vi "common_GUI_UpdateDeviceList.vi"(8 "error in (no error)":errorcluster, 9 "Controls[]":refnum<vi>[](array[refnum]), 10 "Arguments":string, 11 "SQL Server Info":T2) -> (0 "error out":errorcluster)   [LabVIEW 2013]
uses:
  Shared/MySQL/typedefs/mysql_authentication.ctl
panel:
  out "Array":string[](array[string])
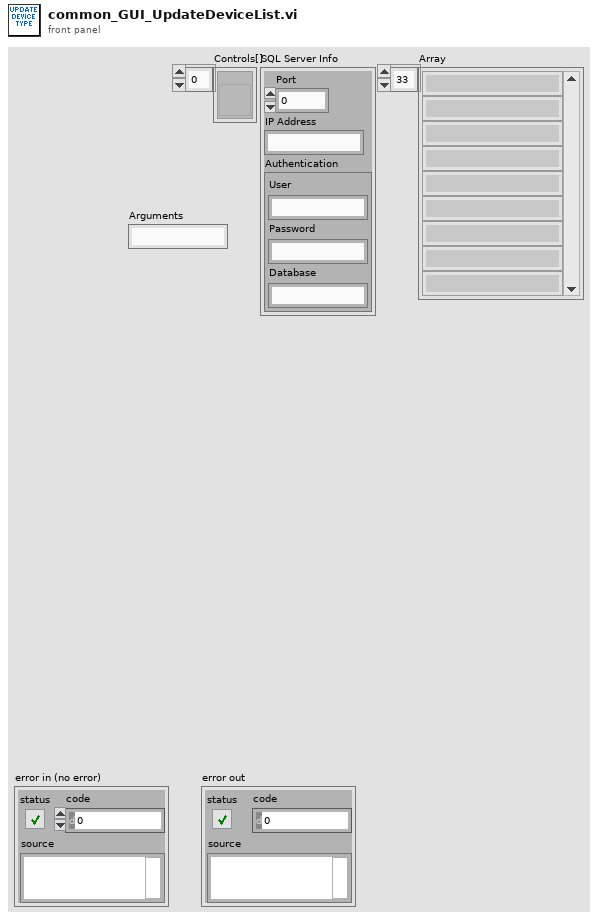
[diagram p1: front panel]
types:
  T1 = typedef "mysql_authentication.ctl" = cluster{"User":string, "Password":string, "Database":string}
  T2 = cluster{"Port":u16, "IP Address":string, "Authentication":T1}
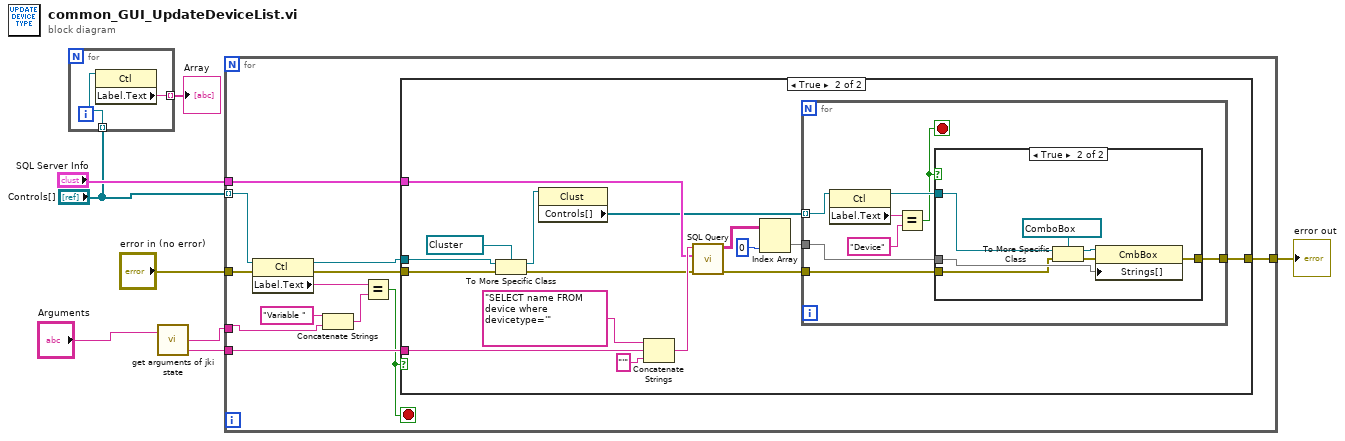
[diagram p0: block diagram]
diagram:
  n1 = for {
    tunnel: "Controls[]" -> [w10] mode=indexing
    tunnel: [w9] -> w1 mode=indexing
    n2 = property class="Ctl"(reference=w10) -> ("Label.Text"=w9:string)  [unwired: 1 in, 2 out]
  }
  "Array" <- w1
  n3 = call "get arguments of jki state.vi"("jki arguments"="Arguments") -> ("Arg 1"=w7:string, "Arg 2"=w8:string)  [unwired: 1 in, 1 out]
  n4 = for {
    tunnel: "Controls[]" -> [w22] mode=indexing
    tunnel: w7 -> [w12]
    tunnel: "error in (no error)" -> [w18]
    tunnel: "SQL Server Info" -> [w17]
    tunnel: [w16] -> w5
    tunnel: w8 -> [w15]
    stop <- w14 stop-if-true
    n5 = property class="Ctl"(reference=w22, error in=w18) -> (reference out=w20:refnum<vi>, error out=w19:errorcluster, "Label.Text"=w21:string)
    n6 = Concatenate Strings("Variable ", w12) -> (w11:string)
    n7 = Equal?(x=w21, y=w11) -> (x = y?=w14:bool)
    n8 = case shown="True" w14 {
      tunnel: w20 -> [_ w26]
      tunnel: w19 -> [w23 w38]
      tunnel: w15 -> [_ w32]
      tunnel: w17 -> [_ w30]
      tunnel: [w23 w27] -> w16
      frame False {
      }
      frame True {
        n9 = To More Specific Class(target class=refnum<vi> refnum ("Device 2"), reference=w26, error in=w38) -> (specific class reference=w25:refnum<vi>, error out=w29:errorcluster)
        n10 = property class="Clust"(reference=w25) -> ("Controls[]"=w24:refnum<vi>[])  [unwired: 1 in, 2 out]
        n11 = Concatenate Strings("SELECT name FROM device where devicetype='" ("Query"), w32, "'" ("string")) -> (w33:string)
        n12 = call "SQL Query.vi"("error in (no error)"=w29, "SQL Server Info"=w30, "Query"=w33) -> ("error out"=w28:errorcluster, "data"=w37:string[][])  [unwired: 7 in]
        n13 = Index Array(array=w37, index (col)=0 ("disabled index (col)")) -> (element=w31:string[])  [unwired: 1 in]
        n14 = for {
          tunnel: w31 -> [w47]
          tunnel: w28 -> [w46]
          tunnel: [w45] -> w27
          tunnel: w24 -> [w43] mode=indexing
          stop <- w40 stop-if-true
          n15 = property class="Ctl"(reference=w43) -> (reference out=w42:refnum<vi>, "Label.Text"=w41:string)  [unwired: 1 in, 1 out]
          n16 = Equal?(x=w41, y="Device") -> (x = y?=w40:bool)
          n17 = case shown="True" w40 {
            tunnel: w47 -> [_ w55]
            tunnel: w46 -> [w48 w50]
            tunnel: [w48 w51] -> w45
            tunnel: w42 -> [_ w53]
            frame False {
            }
            frame True {
              n18 = To More Specific Class(target class=refnum<vi> refnum ("Device 2"), reference=w53, error in=w50) -> (specific class reference=w52:refnum<vi>, error out=w49:errorcluster)
              n19 = property class="CmbBox"(reference=w52, error in=w49, "Strings[]"=w55) -> (error out=w51:errorcluster)  [unwired: 1 out]
            }
          }
        }
      }
    }
  }
  "error out" <- w5
